vi "read_all_uploadDB.vi"(2 "error in (no error)":errorcluster, 3 "Folder Path":path) -> (0 "error out":errorcluster, 1 "All Files in Dir":path[](array[path]))   [LabVIEW 2017]
panel:
  out "Processed file name":path
  out "File Num":i32
  out "Datasets Num":i32
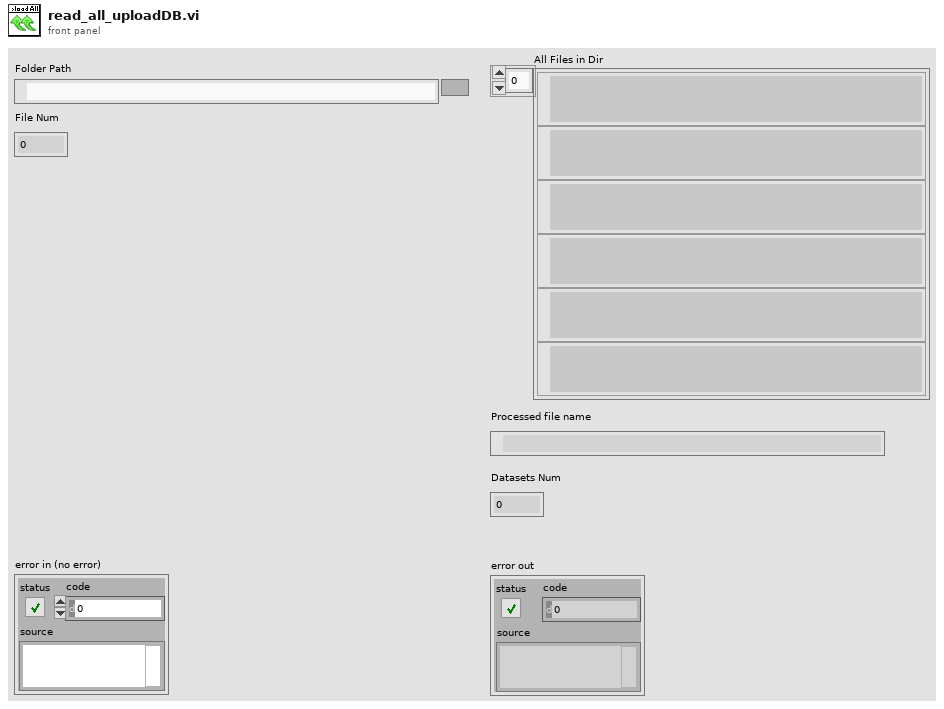
[diagram p1: front panel]
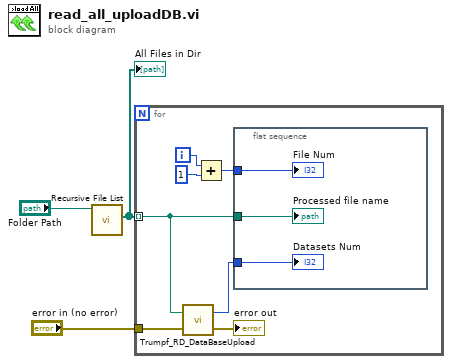
[diagram p0: block diagram]
diagram:
  n1 = call <vilib>:"Recursive File List.vi"("Folder Path"="Folder Path") -> ("All Files in Dir"=w2:path[])  [unwired: 6 in, 4 out]
  "All Files in Dir" <- w2
  n2 = for {
    tunnel: w2 -> [w4] mode=indexing
    tunnel: "error in (no error)" -> [w10]
    i -> [w7]
    n3 = call "Trumpf_RD_DataBaseUpload.vi"("error in (no error)"=w10, "Bar_LIV_Data"=w4) -> ("error out"=→"error out":errorcluster, "Datasets Num"=w8:i32)
    n4 = Add(x=w7, y=1) -> (x+y=w5:i32)
    n5 = flat-sequence {
      tunnel: w8 -> [w13]
      tunnel: w5 -> [w12]
      tunnel: w4 -> [w11]
      frame #0 {
        "Datasets Num" <- w13
        "File Num" <- w12
        "Processed file name" <- w11
      }
    }
  }
